vi "Write to DB as list.vi"(8 "error in (no error)":errorcluster, 11 "Database Entry in":refnum<class "Database Entry.lvclass">) -> (0 "error out":errorcluster, 2 "Stack names":string[](array[string]), 3 "Database Entry out":refnum<class "Database Entry.lvclass">)   [LabVIEW 2021, in "Database Entry.lvclass"]
uses:
  Database Entry.lvclass
  Database Entry.lvclass/Database Entry.ctl
  <vilib>/Utility/file.llb/Read Delimited Spreadsheet (string).vi
  <vilib>/Utility/file.llb/Write Delimited Spreadsheet (string).vi
  Components/Stack/Stack.lvclass
panel:
  out "Strings out":string[](array[string])
  out "Data cluster":T1={"module or proto"="proto", " geometry"="full", "resolution"="LD", "baselayer"="BA_123", "toplayer"="SI_789", "bl_pos"="1", "tl_pos"="1", "put_pos"="1", "region"="1", "asstray"="1", "comptray"="1", "put"="1", "date"="2024-04-02", "timestart"="1:12:12.442", "timeend"="1:23:45.244", "operator"="cmuperson", "tape"="some", "glue"="some", "stack name"="some", "Adhesive type"="", "Comments"="", "Temperature"="", "Relative Humidity"="", "Sensor grade"="", "ROC version"="", "Baseplate material"=""}
  out "error out py":errorcluster
  in  "error in (no error) py":errorcluster
  # "Debug instructions\n#### The order of values in db_data_cols must match the order of values in Data cluster in Stack.lvclass: Get stack data.vi \n#### The variable names below correspond to postgres col name. LV does not neet to match the col numes but just the values. \n#### Right-click on the Data cluster on the front panel and click on 'reorder controls' to verify the order is correct in the code. \n#### The physical position of the fields is different from the actual position.\n\nIn Main VIs/python_db/postgres_tools.py, see functions 'assembly_data' and 'assembly_data_as_list'."
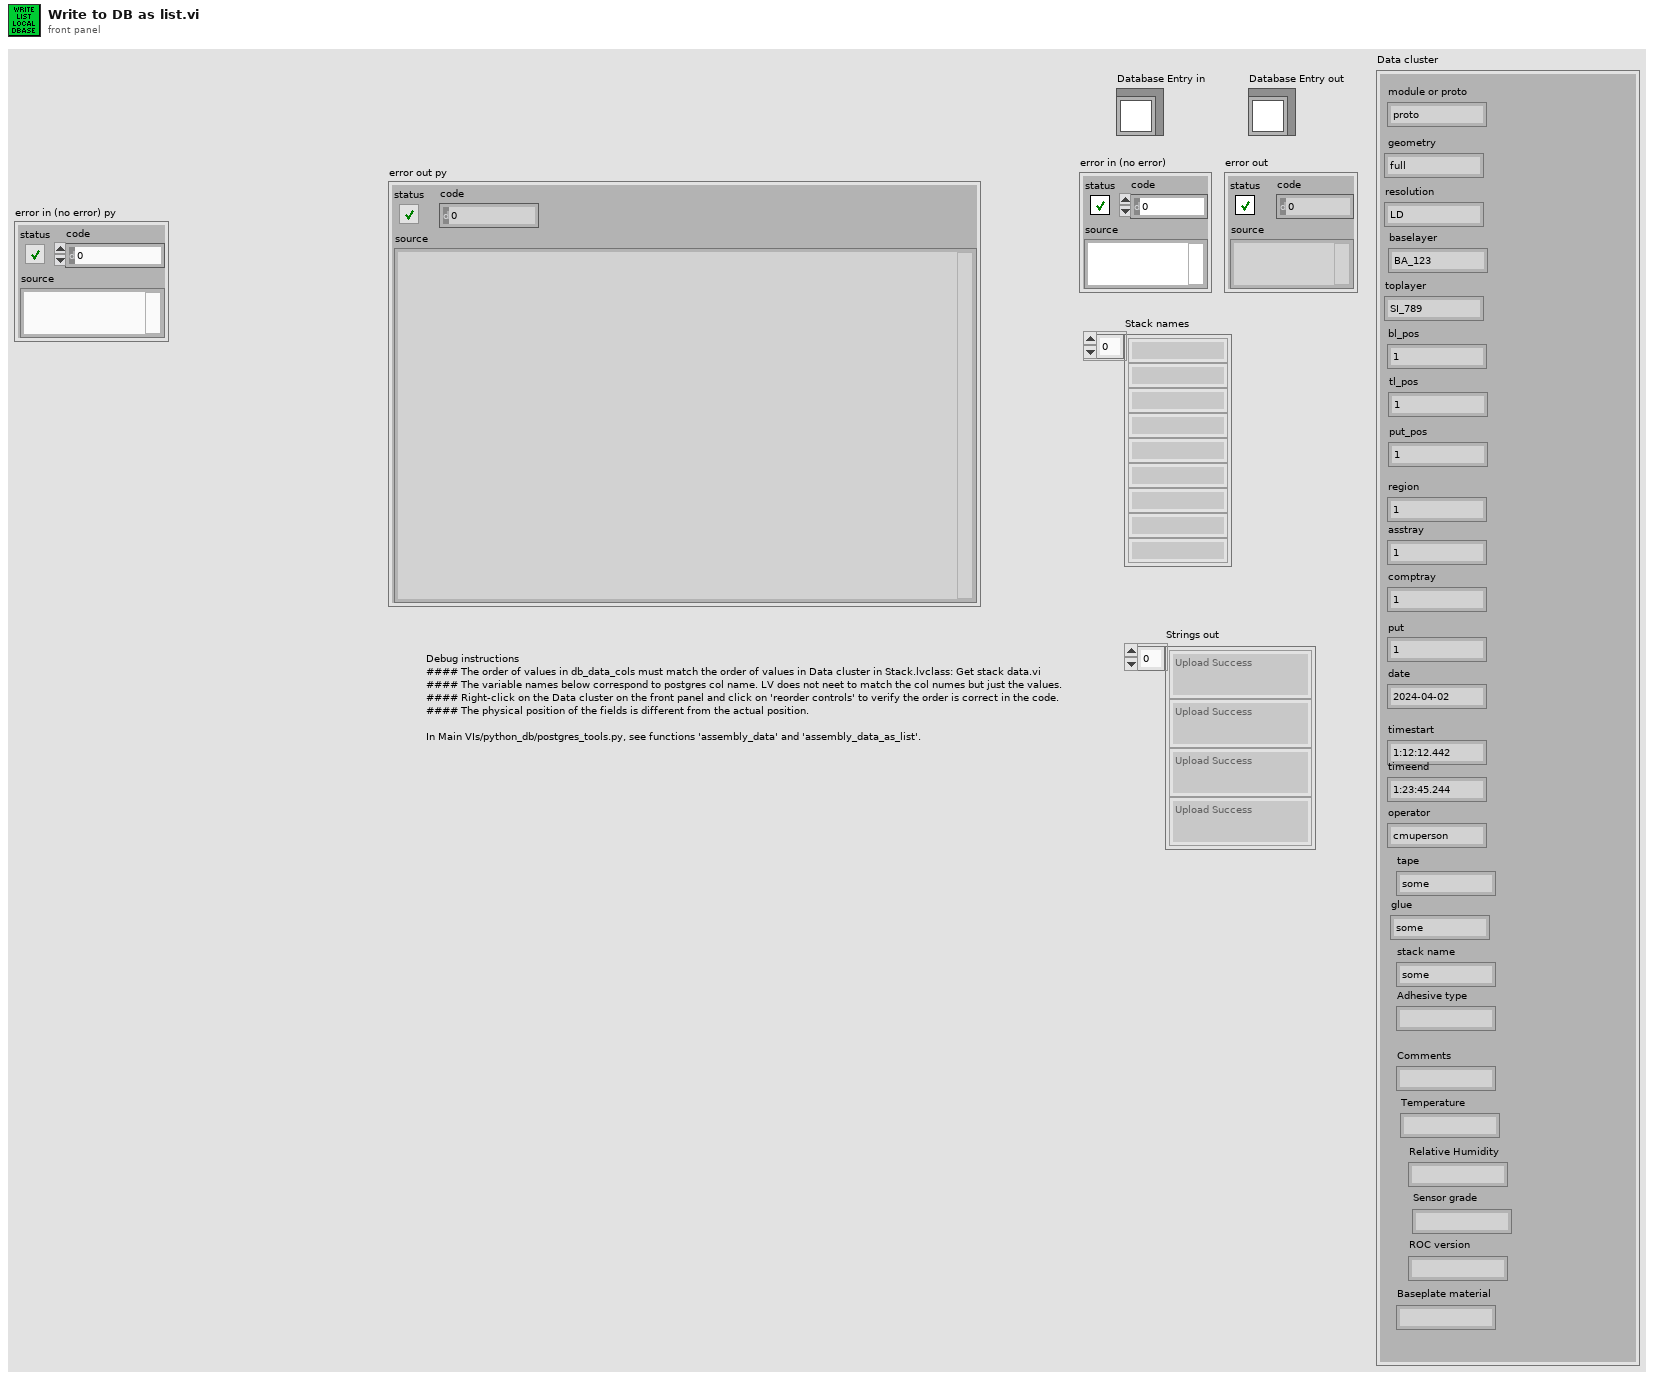
[diagram p1: front panel]
types:
  T1 = cluster{"module or proto":string, " geometry":string, "resolution":string, "baselayer":string, "toplayer":string, "bl_pos":string, "tl_pos":string, "put_pos":string, "region":string, "asstray":string, "comptray":string, "put":string, "date":string, "timestart":string, "timeend":string, "operator":string, "tape":string, "glue":string, "stack name":string, "Adhesive type":string, "Comments":string, "Temperature":string, "Relative Humidity":string, "Sensor grade":string, "ROC version":string, "Baseplate material":string}
  T2 = typedef "File Paths.ctl" = cluster{"Glue Pattern Folder":path, "Carrier Tray Folder":path, "Pick Up Tool Fixture Folder":path, "Components Folder":path, "Bellows Tool Offset.txt":path, "Pick Up Tool Offset.txt":path, "Dispense Tip Offset.txt":path, "Log Files":path, "Gantry Assembly Map.txt":path, "Syringe and offset map.txt":path, "Controllers Folder":path, "Local dbase config":path}
  T3 = cluster{"type (proto/module)":string, " geometry":string, "resolution":string, "baselayer":string, "toplayer":string, "bl_pos":string, "tl_pos":string, "put_pos":string, "region":string, "asstray":string, "comptray":string, "put":string, "date":string, "timestart":string, "timeend":string, "operator":string, "tape":string, "glue":string, "stack name":string, "Adhesive type":string, "Comments":string, "Temperature":string, "Relative Humidity":string, "Sensor grade":string, "ROC version":string, "Baseplate material":string}
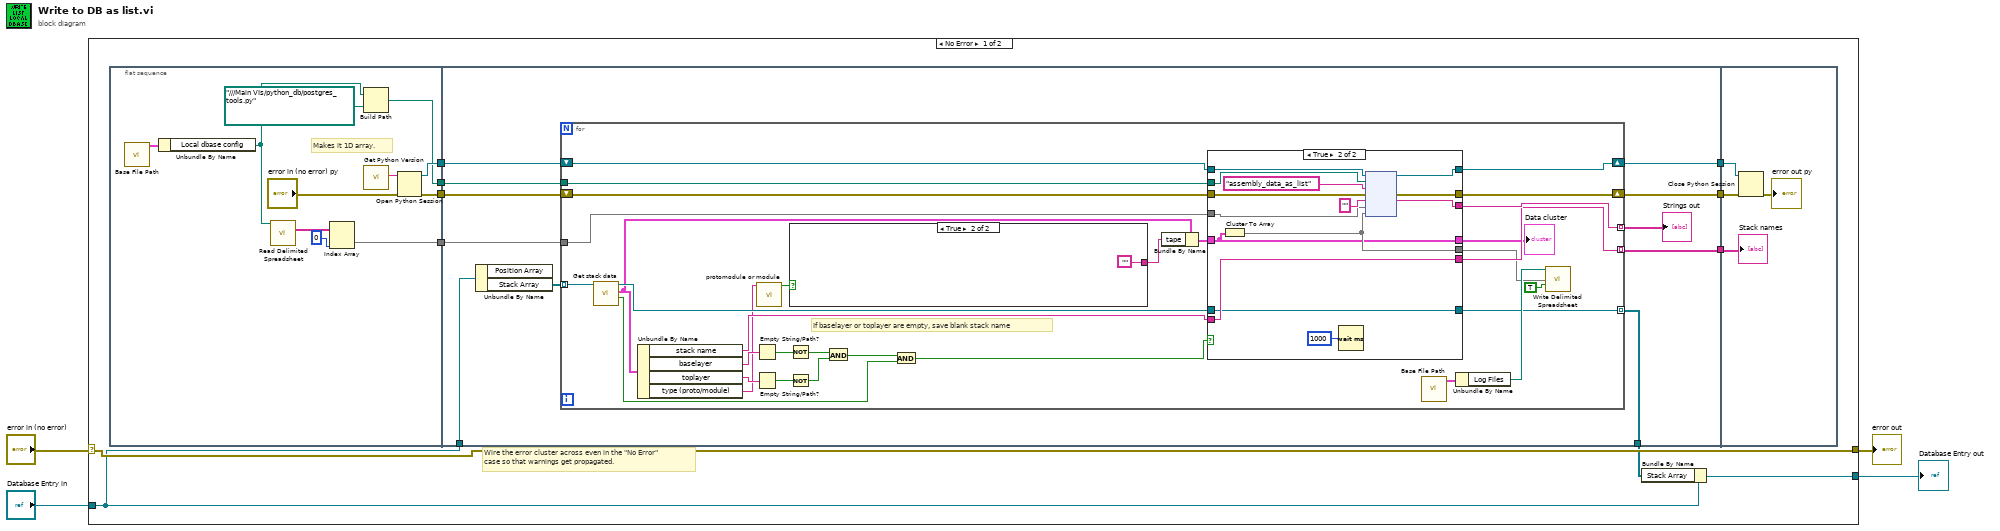
[diagram p0: block diagram]
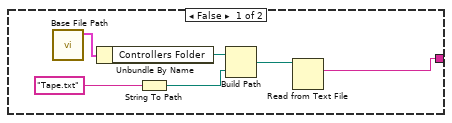
[diagram p2: hidden frame]
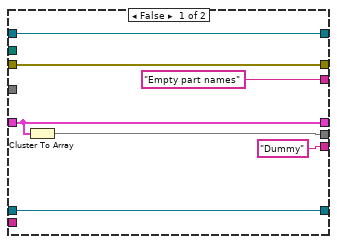
[diagram p3: hidden frame]
diagram:
  n1 = case shown="No Error" "error in (no error)" {
    selector: "error in (no error)" -> [w15 w102]
    tunnel: [w15 w102] -> w3
    tunnel: [w7 w101] -> w1
    tunnel: "Database Entry in" -> [w6 w101]
    frame No Error {
      # "Wire the error cluster across even in the \"No Error\"\ncase so that warnings get propagated."
      n2 = flat-sequence {
        tunnel: [w25] -> w14
        tunnel: [w26] -> w13
        tunnel: [w22] -> w12
        tunnel: [w18] -> w11
        tunnel: [w36] -> w10
        tunnel: [w35] -> w9
        tunnel: w14 -> [w37]
        tunnel: w13 -> [w34]
        tunnel: w12 -> [w33]
        tunnel: w11 -> [w32]
        tunnel: w6 -> [w31]
        tunnel: [w29] -> w8
        tunnel: [w28] -> w5
        tunnel: w10 -> [w99]
        tunnel: w9 -> [w100]
        tunnel: w8 -> [w97]
        frame #0 {
          # "Makes it 1D array."
          n3 = call "Base File Path.vi"() -> ("Paths Out"=w23:T2)  [unwired: 11 in]
          n4 = Unbundle By Name(w23) -> ("Local dbase config"=w21:path)
          n5 = call-poly <vilib>:"Read Delimited Spreadsheet.vi"("file path (dialog if empty)"=w21) -> ("all rows"=w20:string[][])  [unwired: 9 in, 5 out]
          n6 = Index Array(array=w20, index (col)=0 ("disabled index (col)")) -> (element=w18:string[])  [unwired: 1 in]
          n7 = Build Path(base path=w21, name or relative path=path "../../../Main VIs/python_db/postgres_tools.py" ("module path")) -> (appended path=w22:path)
          n8 = call "Get Python Version.vi"() -> ("Python Version"=w16:string)  [unwired: 10 in, 1 out]
          n9 = Open Python Session(python version=w16, 3:"error in (no error) py") -> (session out=w26:refnum<k35>, error out=w25:errorcluster)  [unwired: 1 in]
        }
        frame #1 {
          n10 = Unbundle By Name(w31) -> ("Stack Array"=w30:refnum<class "Stack.lvclass">[])  [unwired: 1 out]
          n11 = for {
            tunnel: w33 -> [w60]
            shift-right: [w68] -> w36
            shift-left: w37 -> [w59]
            shift-right: [w67] -> w35
            shift-left: w34 -> [w61]
            tunnel: [w66] -> w27 mode=indexing
            tunnel: w30 -> [w65] mode=indexing
            tunnel: w32 -> [w62]
            tunnel: [w58] -> w29 mode=indexing
            tunnel: [w51] -> w28 mode=indexing
            # "If baselayer or toplayer are empty, save blank stack name"
            n12 = call "Get stack data.vi"("Stack in"=w65) -> ("Is real run"=w45:bool, "Data cluster"=w42:T3, "Stack out"=w56:refnum<class "Stack.lvclass">)  [unwired: 7 in, 1 out]
            n13 = Unbundle By Name(w42) -> ("stack name"=w55:string, "baselayer"=w54:string, "toplayer"=w53:string, "type (proto/module)"=w41:string)
            n14 = Empty String/Path?(string/path=w54) -> (empty?=w49:bool)
            n15 = Empty String/Path?(string/path=w53) -> (empty?=w47:bool)
            n16 = call "protomodule or module.vi"("assembly type"=w41) -> ("protomodule? (T)"=w40:bool)  [unwired: 10 in]
            n17 = Not(x=w49) -> (.not. x?=w48:bool)
            n18 = Not(x=w47) -> (.not. x?=w46:bool)
            n19 = case shown="True" w40 {
              tunnel: [w69 ""] -> w39
              frame False {
                n20 = call "Base File Path.vi"() -> ("Paths Out"=w74:T2)  [unwired: 11 in]
                n21 = Unbundle By Name(w74) -> ("Controllers Folder"=w73:path)
                n22 = String To Path(string="Tape.txt") -> (path=w71:path)
                n23 = Build Path(base path=w73, name or relative path=w71) -> (appended path=w70:path)
                n24 = Read from Text File(file (use dialog)=w70) -> (text=w69:string)  [unwired: 3 in, 3 out]
              }
              frame True {
              }
            }
            n25 = And(x=w48, y=w46) -> (x .and. y?=w44:bool)
            n26 = And(x=w44, y=w45) -> (x .and. y?=w43:bool)
            n27 = Bundle By Name(cluster=w42, "tape"=w39) -> (w38:T3)
            n28 = case shown="True" w43 {
              tunnel: [w81 w96] -> w68
              tunnel: [w82 w95] -> w67
              tunnel: ["Empty part names" w94] -> w66
              tunnel: w62 -> [_ w92]
              tunnel: w61 -> [w82 w91]
              tunnel: w60 -> [_ w90]
              tunnel: w59 -> [w81 w89]
              tunnel: w55 -> [_ w87]
              tunnel: ["Dummy" ("stack name") w87] -> w58
              tunnel: w38 -> [w76 w84]
              tunnel: [w77 w85] -> w52
              tunnel: w56 -> [w78 w86]
              tunnel: [w78 w86] -> w51
              tunnel: [w76 w84] -> w50
              frame False {
                n29 = Cluster To Array(cluster=w76) -> (array=w77:string[])
              }
              frame True {
                n30 = Cluster To Array(cluster=w84) -> (array=w85:string[])
                n31 = Wait (ms)(milliseconds to wait=u32 1000) -> ()  [unwired: 1 out]
                n32 = node(w91, w90, "assembly_data_as_list" ("function name"), w89, "", w92, w85) -> (w95:refnum<k35>, w96:errorcluster, w94:string)  [unwired: 2 in, 2 out]
              }
            }
            "Data cluster" <- w50
            n33 = call "Base File Path.vi"() -> ("Paths Out"=w64:T2)  [unwired: 11 in]
            n34 = Unbundle By Name(w64) -> ("Log Files"=w63:path)
            n35 = call-poly <vilib>:"Write Delimited Spreadsheet.vi"("file path (dialog if empty)"=w63, "1D data"=w52, "append to file? (new file:F)"=TRUE) -> ()  [unwired: 11 in, 2 out]
          }
          "Strings out" <- w27
        }
        frame #2 {
          n36 = Close Python Session(session in=w100, error in=w99) -> (11:→"error out py":errorcluster)
          "Stack names" <- w97
        }
      }
      n37 = Bundle By Name(cluster=w6, "Stack Array"=w5) -> (w7:refnum<class "Database Entry.lvclass">)
    }
    frame Error {
    }
  }
  "error out" <- w3
  "Database Entry out" <- w1
